vi "Buffer Base Timestamp.vi"(8 "error in (no error)":errorcluster, 9 "Buffer Name":string, 11 "VISA resource name":refnum<visa-resource-name>) -> (0 "error out":errorcluster, 1 "Base Time Stamp (s)":dbl, 3 "VISA resource name out":refnum<visa-resource-name>, 4 "Command String":string)   [LabVIEW 2018, in "Keithley 2600 Series.lvlib"]
doc: "This VI gets the base timestamp of the reading buffer.\n\nThe base timestamp is the time when the first reading was stored from time of power-up.\n\n<b>Functions and Attributes Used</b>\n<buffername>.basetimestamp"
uses:
  Keithley 2600 Series.lvlib
  Private/GlobalVariables.vi
panel:
  # "(c) 2008 Keithley Instruments, Inc.  ALL RIGHTS RESERVED."
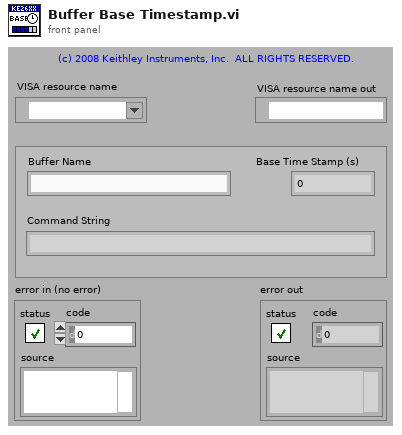
[diagram p1: front panel]
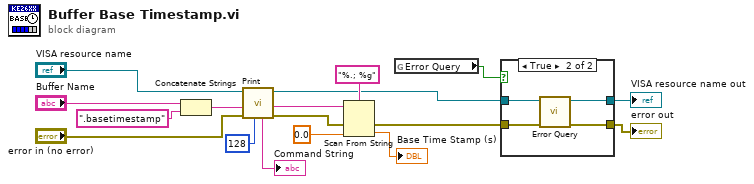
[diagram p0: block diagram]
diagram:
  n1 = Concatenate Strings("Buffer Name", ".basetimestamp" ("command")) -> (w8:string)
  n2 = call "Print.vi"("Byte Count (1024)"=u32 128, "error in (no error)"="error in (no error)", "Input"=w8, "VISA resource name"="VISA resource name") -> ("error out"=w4:errorcluster, "Output"=w5:string, "VISA resource name out"=w1:refnum<visa-resource-name>, "Command String"=→"Command String":string)  [unwired: 1 in, 3 out]
  n3 = Scan From String(format string="%.; %g", input string=w5, error in=w4, default 1=0.0 ("default value 1")) -> (error out=w12:errorcluster, output 1=→"Base Time Stamp (s)":dbl)  [unwired: 1 in, 2 out]
  n4 = global read "GlobalVariables.vi" "Error Query"() -> (w13:bool)
  n5 = case shown="True" w13 {
    tunnel: w12 -> [w19 w23]
    tunnel: [w18 w22] -> w11
    tunnel: [w19 w21] -> w10
    tunnel: w1 -> [w18 w20]
    frame False {
    }
    frame True {
      n6 = call "Error Query.vi"("error in (no error)"=w23, "VISA resource name"=w20) -> ("error out"=w21:errorcluster, "VISA resource name out"=w22:refnum<visa-resource-name>)  [unwired: 8 out]
    }
  }
  "VISA resource name out" <- w11
  "error out" <- w10
